vi "RunCode.vi"(2 "SubPanel in":refnum<vi>, 3 "Code name":string) -> ()   [LabVIEW 2012]
panel:
  out "Execution:State":T1(ring)
  out "error out":errorcluster
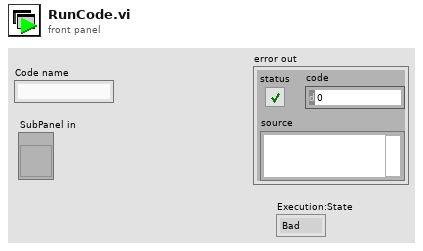
[diagram p1: front panel]
types:
  T1 = enum32{"Bad", "Idle", "Run top level", "Running"}
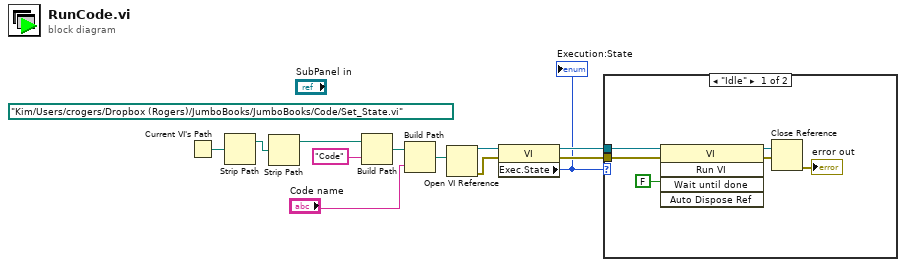
[diagram p0: block diagram]
diagram:
  (unwired) path "/Kim/Users/crogers/Dropbox (Rogers)/JumboBooks/JumboBooks/Code/Set_State.vi" ("vi path")
  n1 = Current VI's Path() -> (path=w9:path)
  n2 = Strip Path(path=w9) -> (stripped path=w8:path)  [unwired: 1 out]
  n3 = Strip Path(path=w8) -> (stripped path=w7:path)  [unwired: 1 out]
  n4 = Build Path(base path=w7, name or relative path="Code") -> (appended path=w11:path)
  n5 = Build Path(base path=w11, name or relative path="Code name") -> (appended path=w1:path)
  n6 = Open VI Reference(vi path=w1) -> (vi reference=w5:refnum<vi>, error out=w6:errorcluster)  [unwired: 5 in]
  n7 = property class="VI"(reference=w5, error in=w6) -> (reference out=w4:refnum<vi>, error out=w3:errorcluster, "Exec.State"=w2:T1)
  "Execution:State" <- w2
  n8 = case shown="\"Idle\"" w2 {
    tunnel: w4 -> [w14 _]
    tunnel: w3 -> [w15 _]
    frame "Idle" {
      n9 = invoke class="VI" method="Run VI"(reference=w14, error in=w15, "Wait until done"=FALSE ("ShowHScrollBar")) -> (reference out=w18:refnum<vi>, error out=w16:errorcluster)  [unwired: 2 in, 3 out]
      n10 = Close Reference(reference=w18, error in (no error)=w16) -> (error out=→"error out":errorcluster)
    }
    frame Default {
    }
  }
